vi "task_msgUserEvent.vi"(8 "error in (no error)":errorcluster, 10 "taskChannel":refnum<class "ITaskChannel.lvclass">, 11 "ITask in":refnum<class "ITask.lvclass">) -> (0 "error out":errorcluster, 3 "ITask out":refnum<class "ITask.lvclass">)   [LabVIEW 2023]
uses:
  TLC_Daemon.lvlib
  ITask/ITask.lvclass
  ITaskChannel/ITaskChannel.lvclass
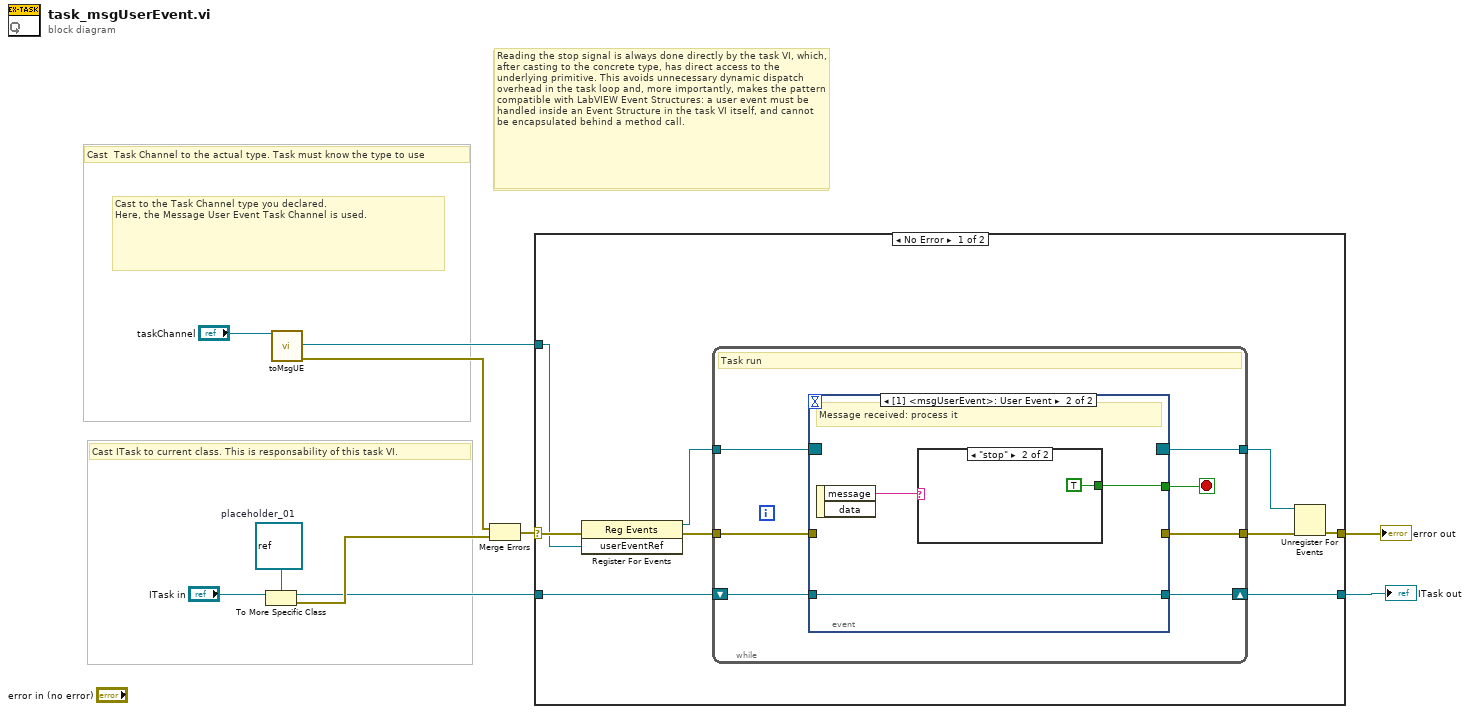
[diagram p0: block diagram]
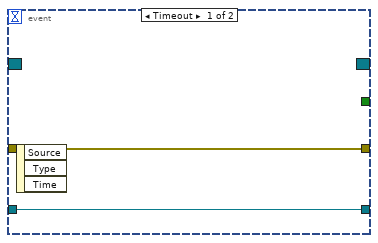
[diagram p2: hidden frame]
diagram:
  w7 = refnum<class> refnum  # placeholder_01
  # "Cast to the Task Channel type you declared.\nHere, the Message User Event Task Channel is used."
  # "The stop signal is always handled directly by the task VI, which, after casting to the concrete type, has direct access to the underlying primitive. This avoids unnecessary dynamic dispatch overhead in the task loop and, more importantly, makes the pattern compatible with LabVIEW Event Structures: a user event must be handled inside an Event Structure in the task VI itself, and cannot be encapsulated behind a method call."
  # "Reading the stop signal is always done directly by the task VI, which, after casting to the concrete type, has direct access to the underlying primitive. This avoids unnecessary dynamic dispatch overhead in the task loop and, more importantly, makes the pattern compatible with LabVIEW Event Structures: a user event must be handled inside an Event Structure in the task VI itself, and cannot be encapsulated behind a method call."
  # "Cast ITask to current class. This is responsability of this task VI."
  # "Cast  Task Channel to the actual type. Task must know the type to use"
  n1 = To More Specific Class(target class=w7, reference="ITask in") -> (specific class reference=w3:refnum<class>, error out=w8:errorcluster)  [unwired: 1 in]
  n2 = call "toMsgUE.vi"("ITaskChannel"="taskChannel") -> ("error out"=w6:errorcluster, "userEventRef"=w1:refnum<user-event>)  [unwired: 9 in]
  n3 = Merge Errors(w6, w8) -> (w5:errorcluster)
  n4 = case shown="No Error" w5 {
    selector: w5 -> [w19 w34]
    tunnel: w1 -> [w13 _]
    tunnel: [w12 w33] -> w2
    tunnel: [w15 w34] -> w4
    tunnel: w3 -> [w11 w33]
    frame No Error {
      n5 = register-events(error in=w19, w13) -> (reference out=w17:refnum<event-registration>, error out=w18:errorcluster)  [unwired: 1 in]
      n6 = while {
        tunnel: w18 -> [w26]
        tunnel: [w25] -> w14
        tunnel: w17 -> [w24]
        tunnel: [w22] -> w16
        shift-right: [w20] -> w12
        shift-left: w11 -> [w21]
        stop <- w23 stop-if-true
        # "Task run"
        n7 = event shown="[1] <msgUserEvent>: User Event" {
          selector: w24 -> [_ _]
          dyn-events: [_ _] -> w22
          timeout: _ -> [_ _]
          tunnel: w26 -> [w28 _]
          tunnel: [w28 _] -> w25
          tunnel: [_ w30] -> w23
          tunnel: w21 -> [w27 w29]
          tunnel: [w27 w29] -> w20
          event Timeout {
            n8 = event-data() -> ()  [unwired: 1 in, 3 out]
          }
          event User Event {
            # "Message received: process it"
            n9 = event-data() -> ("message"=w31:string)  [unwired: 1 in, 1 out]
            n10 = case shown="\"stop\"" w31 {
              tunnel: [_ TRUE] -> w30
              frame Default {
              }
              frame "stop" {
              }
            }
          }
        }
      }
      n11 = Unregister For Events(event registration refnum=w16, error in=w14) -> (error out=w15:errorcluster)
    }
    frame Error {
    }
  }
  "error out" <- w4
  "ITask out" <- w2
